vi "EloMec Tester.vi"() -> ()   [LabVIEW 2017]
uses:
  Core/AI Robot.ctl
  Intel/Functions Enum.ctl
  Intel/AttackerStates.ctl
  Path Planning/RRT/PathDests.ctl
  Path Planning/RRT/PathDest.ctl
  <vilib>/Instr/_visa.llb/VISA Configure Serial Port (Instr).vi
panel:
  out "appended array":T1[](array[typedef])
  in  "IDs":u32[](array[numeric])
  in  "high kick":bool
  in  "kickspeedz":sgl=100.0
  in  "Teste de\nengrenagem":bool
  in  "drible":bool
  in  "velangular":sgl
  in  "velnormal":sgl
  in  "veltangent":sgl
  in  "kick":bool
  in  "kickspeedx":sgl=100.0
  out "Numeric 2":dbl
  out "String":string
  out "return count":u32
  in  "stop":bool
  out "string":string
  out "error out":errorcluster
  in  "termination char\n(0xA = '\\n' = LF)":u8=10 format="%.0x"
  in  "VISA resource name":refnum<visa-resource-name>
  in  "Serial Settings":T6={"baud rate"=9600, "data bits"=8, "parity"=enum."None", "stop bits"=10, "flow control"=0} {"flow control" items=["None"=0, "XON/XOFF"=1, "RTS/CTS"=2, "DTR/DSR"=4]; "stop bits" items=["1.0"=10, "1.5"=15, "2.0"=20]; "data bits" min=5 max=8 step=1; "baud rate" items=["75"=75, "110"=110, "134"=134, "150"=150, "300"=300, "600"=600, "1200"=1200, "1800"=1800, "2400"=2400, "4800"=4800, "7200"=7200, "9600"=9600, "14400"=14400, "19200"=19200, "28800"=28800, "38400"=38400, "56000"=56000, "57600"=57600, "115200"=115200, "128000"=128000, "230400"=230400]}
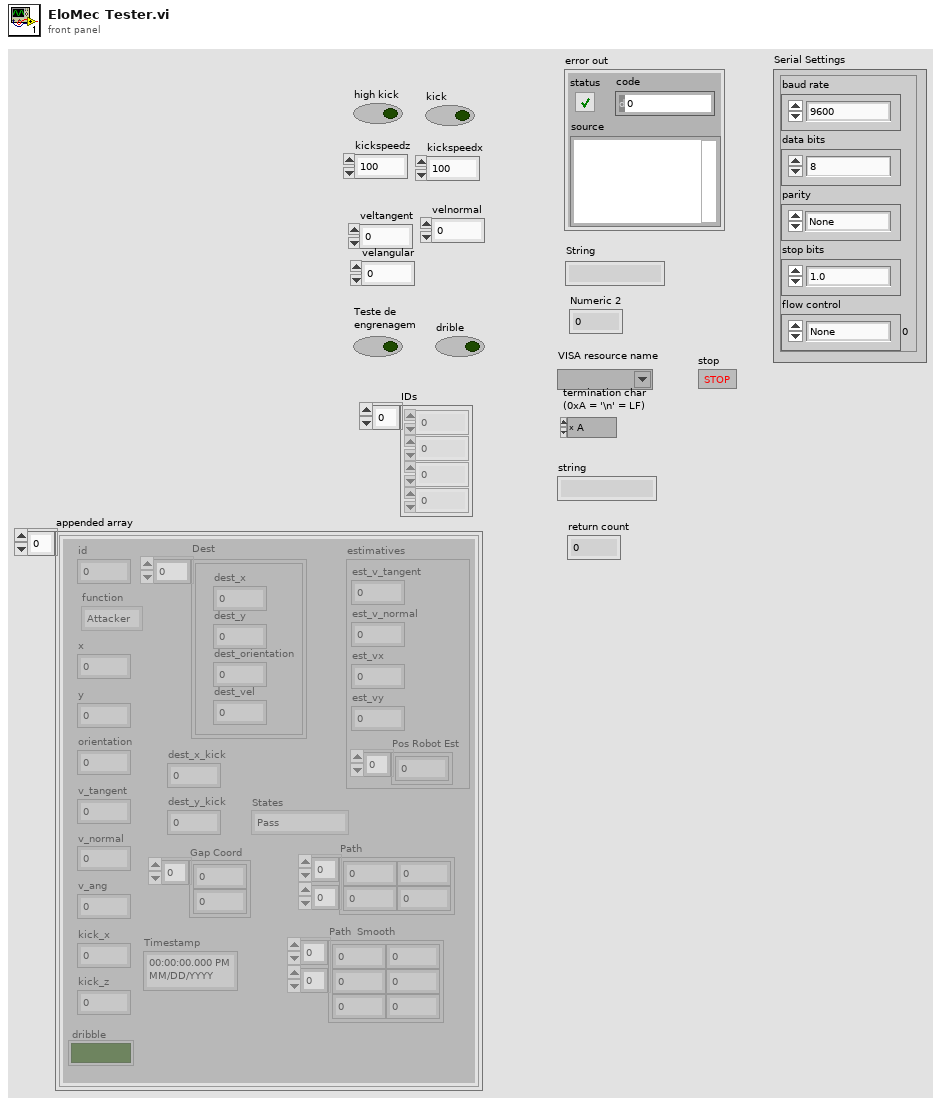
[diagram p1: front panel]
types:
  T1 = typedef "AI Robot.ctl" = cluster{"id":u32, "function":T2, "x":dbl, "y":dbl, "orientation":dbl, "v_tangent":dbl, "v_normal":dbl, "v_ang":dbl, "kick_x":dbl, "kick_z":dbl, "dribble":bool, "Timestamp":timestamp, "estimatives":cluster{"est_v_tangent":dbl, "est_v_normal":dbl, "est_vx":dbl, "est_vy":dbl, "Pos Robot Est":dbl[]}, "dest_x_kick":dbl, "dest_y_kick":dbl, "Gap Coord":dbl[], "States":T3, "Path ":dbl[][], "Path  Smooth":dbl[][], "Dest":T4}
  T2 = typedef "Functions Enum.ctl" = enum16{"Attacker", "Goalie", "Defender", "Striker", "Goto 0", "Dummy", "Kicker", "ZigZag"}
  T3 = typedef "AttackerStates.ctl" = enum16{"Pass", "GoToTangent", "BallGetting", "GoToKick", "Rotate anti-clockwise", "Rotate Clockwise", ""}
  T4 = typedef "PathDests.ctl" = T5[]
  T5 = typedef "PathDest.ctl" = cluster{"dest_x":dbl, "dest_y":dbl, "dest_orientation":dbl, "dest_vel":dbl}
  T6 = cluster{"baud rate":u32, "data bits":u16, "parity":enum16{"None", "Odd", "Even", "Mark", "Space"}, "stop bits":u16, "flow control":u16}
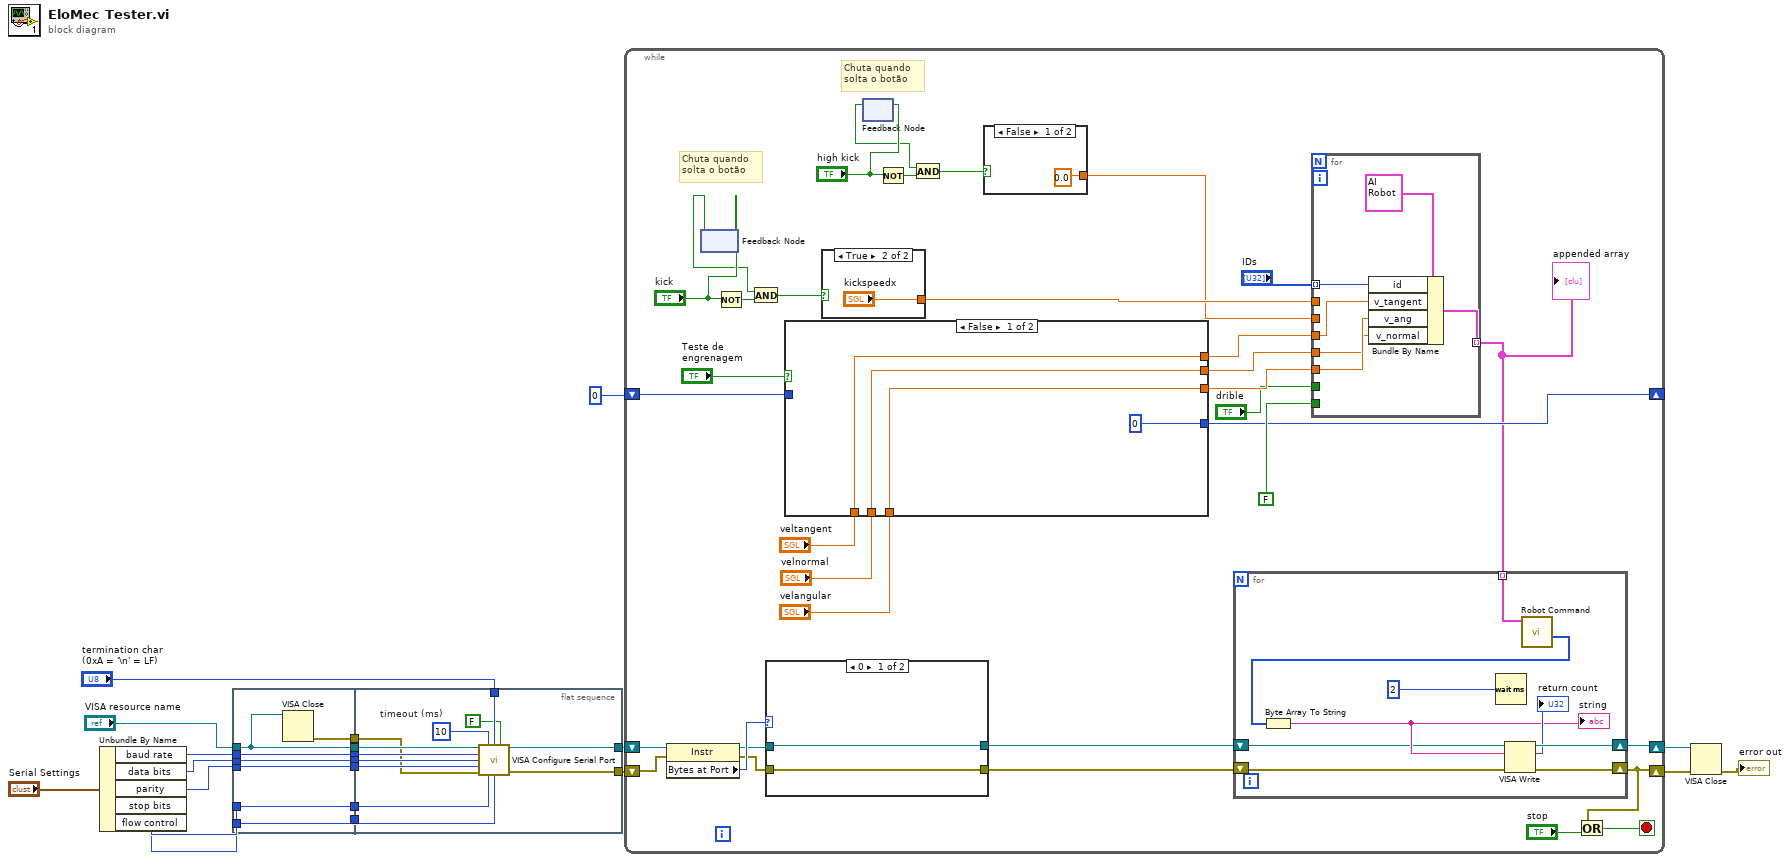
[diagram p0: block diagram]
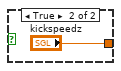
[diagram p2: hidden frame]
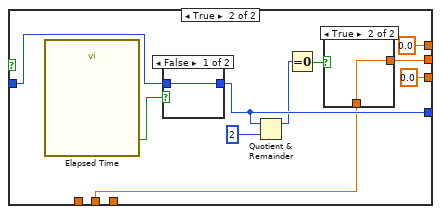
[diagram p3: hidden frame]
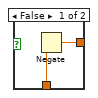
[diagram p4: hidden frame]
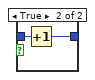
[diagram p5: hidden frame]
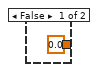
[diagram p6: hidden frame]
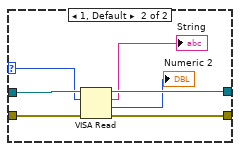
[diagram p7: hidden frame]
diagram:
  n1 = Unbundle By Name("Serial Settings") -> ("baud rate"=w20:u32, "data bits"=w19:u16, "parity"=w18:enum16{"None", "Odd", "Even", "Mark", "Space"}, "stop bits"=w17:u16, "flow control"=w16:u16)
  n2 = flat-sequence {
    tunnel: "VISA resource name" -> [w23]
    tunnel: w16 -> [w24]
    tunnel: w17 -> [w25]
    tunnel: w18 -> [w26]
    tunnel: w19 -> [w27]
    tunnel: w20 -> [w28]
    tunnel: [w28] -> w8
    tunnel: [w27] -> w7
    tunnel: [w26] -> w6
    tunnel: [w25] -> w5
    tunnel: [w24] -> w4
    tunnel: [w23] -> w3
    tunnel: [w22] -> w2
    tunnel: "termination char\n(0xA = '\\n' = LF)" -> [w34]
    tunnel: [w32] -> w13
    tunnel: [w31] -> w11
    tunnel: w8 -> [w40]
    tunnel: w7 -> [w39]
    tunnel: w6 -> [w38]
    tunnel: w5 -> [w37]
    tunnel: w4 -> [w36]
    tunnel: w3 -> [w35]
    tunnel: w2 -> [w29]
    frame #0 {
      n3 = VISA Close(VISA resource name=w23) -> (error out=w22:errorcluster)  [unwired: 1 in]
    }
    frame #1 {
      w30 = u32 10  # timeout (ms)
      n4 = call-poly "VISA Configure Serial Port"("VISA resource name"=w35, "timeout (10sec)"=w30, "termination char\n(0xA = '\\n' = LF)"=w34, "Enable Termination\nChar (T)"=FALSE ("Enable Termination\nChar (T)"), "baud rate (9600)"=w40, "data bits (8)"=w39, "parity (0:none)"=w38, "error in (no error)"=w29, "stop bits (10: 1 bit)"=w37, "flow control (0:none)"=w36) -> ("VISA resource name out"=w32:refnum<visa-resource-name>, "error out"=w31:errorcluster)  [unwired: 4 in]
    }
  }
  n5 = while {
    shift-right: [w74] -> w12
    shift-left: w13 -> [w67]
    shift-right: [w71] -> w10
    shift-left: w11 -> [w66]
    shift-right: [w50] -> _
    shift-left: 0 -> [w51]
    stop <- w72 stop-if-true
    # "Chuta quando \nsolta o botão"
    # "Chuta quando \nsolta o botão"
    n6 = property class="Instr"(reference=w67, error in=w66) -> (reference out=w63:refnum<visa-resource-name>, error out=w64:errorcluster, "Bytes at Port"=w65:u32)
    n7 = feedback #1() -> (w43:bool)  [unwired: 1 in]
    n8 = feedback-in #1("kick") -> ()
    n9 = Not(x="kick") -> (.not. x?=w44:bool)
    n10 = And(x=w43, y=w44) -> (x .and. y?=w61:bool)
    n11 = case shown="0" w65 {
      selector: w65 -> [_ w116]
      tunnel: w64 -> [w114 w122]
      tunnel: [w114 w121] -> w69
      tunnel: w63 -> [w115 w120]
      tunnel: [w115 w119] -> w68
      frame 0 {
      }
      frame 1, Default {
        n12 = VISA Read(VISA resource name=w120, byte count=w116, error in (no error)=w122) -> (VISA resource name out=w119:refnum<visa-resource-name>, read buffer=→"String":string, return count=→"Numeric 2":u32, error out=w121:errorcluster)
      }
    }
    n13 = case shown="False" "Teste de\nengrenagem" {
      tunnel: [w95 sgl 0.0 ("veltangent")] -> w59
      tunnel: "veltangent" -> [w95 _]
      tunnel: [w94 w96] -> w57
      tunnel: "velnormal" -> [w94 w97]
      tunnel: "velangular" -> [w93 _]
      tunnel: [w93 sgl 0.0 ("velangular")] -> w54
      tunnel: w51 -> [_ w102]
      tunnel: [0 w101] -> w50
      frame False {
      }
      frame True {
        n14 = call "Elapsed Time"() -> ("Time has Elapsed"=w105:bool)  [unwired: 12 in, 7 out]
        n15 = case shown="False" w105 {
          tunnel: w102 -> [w109 w111]
          tunnel: [w109 w110] -> w101
          frame False {
          }
          frame True {
            n16 = Increment(x=w111) -> (x+1=w110:i32)
          }
        }
        n17 = Quotient & Remainder(x=w101, y=2) -> (x-y*floor(x/y)=w99:i32)  [unwired: 1 out]
        n18 = Equal To 0?(x=w99) -> (x = 0?=w98:bool)
        n19 = case shown="True" w98 {
          tunnel: w97 -> [w107 w108]
          tunnel: [w106 w108] -> w96
          frame False {
            n20 = Negate(x=w107) -> (-x=w106:sgl)
          }
          frame True {
          }
        }
      }
    }
    n21 = case shown="True" w61 {
      tunnel: [sgl 0.0 ("kickspeedx") "kickspeedx"] -> w62
      frame False {
      }
      frame True {
      }
    }
    n22 = feedback #2() -> (w46:bool)  [unwired: 1 in]
    n23 = feedback-in #2("high kick") -> ()
    n24 = Not(x="high kick") -> (.not. x?=w48:bool)
    n25 = And(x=w46, y=w48) -> (x .and. y?=w49:bool)
    n26 = case shown="False" w49 {
      tunnel: [sgl 0.0 ("kickspeedx") "kickspeedz"] -> w45
      frame False {
      }
      frame True {
      }
    }
    n27 = for {
      tunnel: FALSE -> [_]
      tunnel: w62 -> [_]
      tunnel: w59 -> [w86]
      tunnel: w57 -> [w84]
      tunnel: w54 -> [w85]
      tunnel: "drible" -> [_]
      tunnel: w45 -> [_]
      tunnel: [w89] -> w41 mode=indexing
      tunnel: "IDs" -> [w88] mode=indexing
      n28 = Bundle By Name(cluster=T1 {"id"=0, "function"=enum."Attacker", "x"=0.0, "y"=0.0, "orientation"=0.0, "v_tangent"=0.0, "v_normal"=0.0, "v_ang"=0.0, "kick_x"=0.0, "kick_z"=0.0, "dribble"=FALSE, "Timestamp"=timestamp(0 s since 1904-01-01), "estimatives"={"est_v_tangent"=0.0, "est_v_normal"=0.0, "est_vx"=0.0, "est_vy"=0.0, "Pos Robot Est"=[]}, "dest_x_kick"=0.0, "dest_y_kick"=0.0, "Gap Coord"=[], "States"=enum."Pass", "Path "=[], "Path  Smooth"=[], "Dest"=[]} ("Robot"), "id"=w88, "v_tangent"=w86, "v_ang"=w85, "v_normal"=w84) -> (w89:T1)
    }
    "appended array" <- w41
    n29 = for {
      shift-right: [w81] -> w71
      shift-left: w69 -> [w78]
      shift-right: [w83] -> w74
      shift-left: w68 -> [w77]
      tunnel: w41 -> [w76] mode=indexing
      n30 = Wait (ms)(milliseconds to wait=u32 2) -> ()  [unwired: 1 out]
      n31 = call "Robot Command.vi"("Robot"=w76) -> ("Array"=w75:u8[])  [unwired: 10 in]
      n32 = Byte Array To String(unsigned byte array=w75) -> (string=w79:string)
      "string" <- w79
      n33 = VISA Write(VISA resource name=w77, write buffer=w79, error in (no error)=w78) -> (VISA resource name out=w83:refnum<visa-resource-name>, return count=→"return count":u32, error out=w81:errorcluster)
    }
    n34 = Or(x=w71, y="stop") -> (x .or. y?=w72:bool)
  }
  n35 = VISA Close(VISA resource name=w12, error in (no error)=w10) -> (error out=→"error out":errorcluster)
